vi "VirtualtoRun.vi"(8 "error in (no error)":errorcluster, 10 "VirtualSetup":string, 11 "VirtualOrigin.lvclass In":refnum<class "VirtualOrigin.lvclass">) -> (0 "error out":errorcluster, 2 "VirtualDataArray":refnum<class "VirtualOrigin.lvclass">[](array[class]))   [LabVIEW 2014, in "Project.lvclass"]
uses:
  Project.lvclass
  Virtual/VirtualOrigin.lvclass
  VirtualSetupDataTypeDefine.ctl
  Virtual/Control/AllVirtualTypeData.ctl
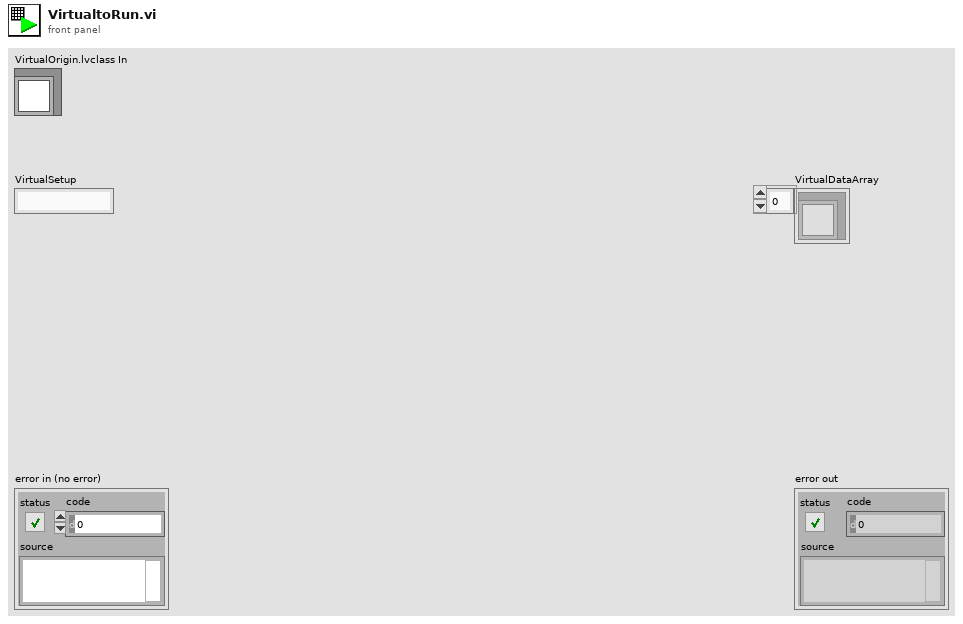
[diagram p1: front panel]
types:
  T1 = typedef "Project.lvclass/VirtualSetupDataTypeDefine.ctl" = T2[]
  T2 = typedef "VirtualOrigin.lvclass/AllVirtualTypeData.ctl" = cluster{"Search Name":string, "Start X":dbl, "Increase X":dbl, "X Step":i32, "Start Y":dbl, "Increase Y":dbl, "Y Step":i32, "Sensor":i32}
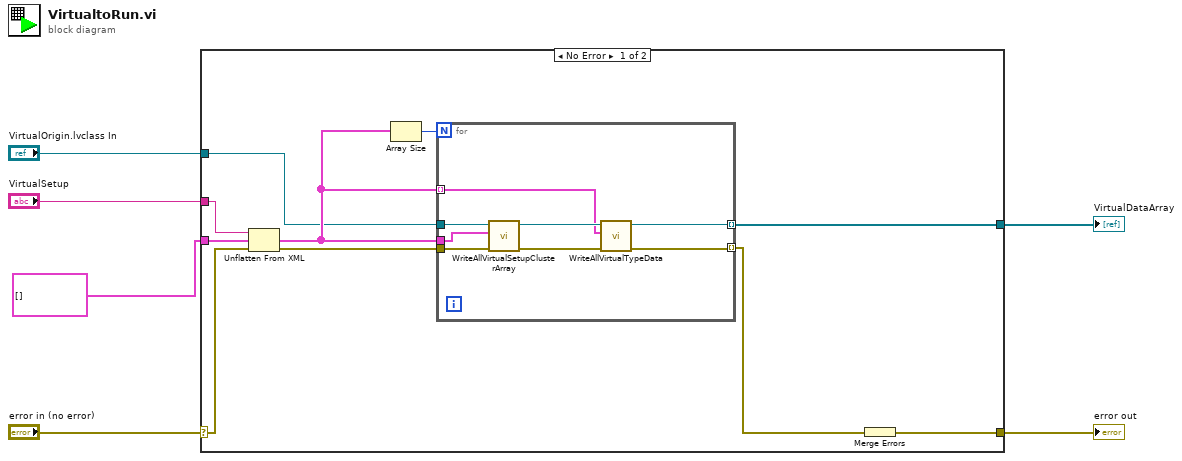
[diagram p0: block diagram]
diagram:
  n1 = case shown="No Error" "error in (no error)" {
    selector: "error in (no error)" -> [w15 w25]
    tunnel: [w11 w25] -> w5
    tunnel: T1 [] ("VirtualSetupClusterArray") -> [w16 _]
    tunnel: "VirtualSetup" -> [w10 _]
    tunnel: "VirtualOrigin.lvclass In" -> [w9 _]
    tunnel: [w7 _] -> w1
    frame No Error {
      n2 = Unflatten From XML(xml string=w10, type=w16, error in (no error)=w15) -> (value=w12:T1, error out=w14:errorcluster)
      n3 = Array Size(array=w12) -> (size(s)=w13:i32)
      n4 = for {
        N: w13 -> [_]
        tunnel: w12 -> [w21] mode=indexing
        tunnel: w14 -> [w24]
        tunnel: w12 -> [w23]
        tunnel: w9 -> [w19]
        tunnel: [w18] -> w7 mode=indexing
        tunnel: [w17] -> w8 mode=indexing
        n5 = call "WriteAllVirtualSetupClusterArray.vi"("error in (no error)"=w24, "VirtualSetupClusterArray In"=w23, "VirtualOrigin.lvclass In"=w19) -> ("error out"=w20:errorcluster, "VirtualOrigin.lvclass Out"=w22:refnum<class "VirtualOrigin.lvclass">)  [unwired: 7 in]
        n6 = call "WriteAllVirtualTypeData.vi"("error in (no error)"=w20, "AllVirtualTypeData In"=w21, "VirtualOrigin.lvclass In"=w22) -> ("error out"=w17:errorcluster, "VirtualOrigin.lvclass Out"=w18:refnum<class "VirtualOrigin.lvclass">)  [unwired: 7 in]
      }
      n7 = Merge Errors(w8) -> (w11:errorcluster)
    }
    frame Error {
    }
  }
  "error out" <- w5
  "VirtualDataArray" <- w1
